vi "Turn (Gyro)(SubVI).vi"(7 "Ang S Up":dbl, 9 "AutoX":dbl, 10 "GyroRef":string="My Gyro RefNum", 11 "DriveMotorRefNum":string="RobotDrive") -> (3 "String":string)   [LabVIEW 2017]
uses:
  <vilib>/Rock Robotics/WPI/SafetyOutput/WPI_SafetyOutputConfigMenu.ctl
  <vilib>/Rock Robotics/WPI/Utilities/WPI_GetSetVariantRefNum.vi
  Robot Global Data.vi
  <vilib>/Rock Robotics/WPI/RobotDrive/WPI_RobotDriveArcadeDrive_Standard(NoSaturation).vi
  <vilib>/Rock Robotics/WPI/RobotDrive/WPI_RobotDriveSafetyCheck.vi
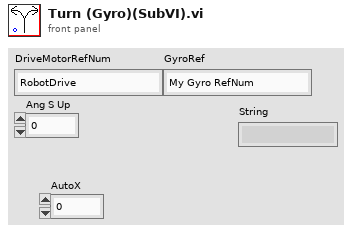
[diagram p1: front panel]
types:
  T1 = typedef "WPI_SafetyOutputConfigMenu.ctl" = enum16{"Enable", "Disable"}
  T2 = typedef "WPI_RobotDriveDevRef.ctl" = cluster{"DevStatus":errorcluster, "Motors[]":T3[], "Square Inputs":bool, "Max Output":dbl}
  T3 = typedef "WPI_MotorControlDeviceRef.ctl" = cluster{"DeviceStatus":errorcluster, "Type":T4, "PWM":cluster{"PWM Channel":T5, "DeadBand":T6}, "CAN":cluster{"Device Number":u8, "SetOutput VI Ref":variant, "GetOutput VI Ref":variant, "Enable VI Ref":variant, "Disable VI Ref":variant, "Data":variant}, "Invert":bool, "DIO PWM":cluster{"PWM \"Enable\" Channel":T5, "DIOChannel":T7, "PWM Rate":dbl}}
  T4 = typedef "WPI_MotorControlType.ctl" = enum16{"PWM", "CAN", "DIO PWM"}
  T5 = typedef "FPGA_DIOPWMChannel.ctl" = enum8{"PWM 0", "PWM 1", "PWM 2", "PWM 3", "PWM 4", "PWM 5", "PWM 6", "PWM 7", "PWM 8", "PWM 9", "PWM MXP 0", "PWM MXP 1", "PWM MXP 2", "PWM MXP 3", "PWM MXP 4", "PWM MXP 5", "PWM MXP 6", "PWM MXP 7", "PWM MXP 8", "PWM MXP 9", "Invalid"}
  T6 = typedef "WPI_PWMDeadband.ctl" = cluster{"Name":string, "maxPositivePwm":i32, "minPositivePwm":i32, "centerPwm":i32, "maxNegativePwm":i32, "minNegativePwm":i32, "angularRange":u16}
  T7 = typedef "FPGA_DIOChannel.ctl" = enum8{"DIO 0", "DIO 1", "DIO 2", "DIO 3", "DIO 4", "DIO 5", "DIO 6", "DIO 7", "DIO 8", "DIO 9", "DIO MXP 0", "DIO MXP 1", "DIO MXP 2", "DIO MXP 3", "DIO MXP 4", "DIO MXP 5", "DIO MXP 6", "DIO MXP 7", "DIO MXP 8", "DIO MXP 9", "DIO MXP 10", "DIO MXP 11", "DIO MXP 12", "DIO MXP 13", "DIO MXP 14", "DIO MXP 15", "SPI Port CS1", "SPI Port CS2", "SPI Port CS3", "SPI Port MISO", "SPI Port MOSI", "Invalid"}
  T8 = typedef "WPI_GyroDevRef.ctl" = cluster{"DevStatus":errorcluster, "Analog Channel":T9, "Gain (VoltsPerDegree/Second)":dbl, "Gyro Type":enum16{"Analog", "XRS450"}, "Handle":i32, "SPI Bus":T10, "Device Found":bool, "Sample Rate":dbl, "Calibrate On Open":bool, "Offset":dbl}
  T9 = typedef "FPGA_AIChannel.ctl" = enum8{"AI 0", "AI 1", "AI 2", "AI 3", "AI MXP 0", "AI MXP 1", "AI MXP 2", "AI MXP 3", "Invalid"}
  T10 = typedef "spi_bus.ctl" = enum16{"SPI On-Board, CS0", "SPI On-Board, CS1", "SPI On-Board, CS2", "SPI On-Board, CS3", "SPI MXP", "Invalid"}
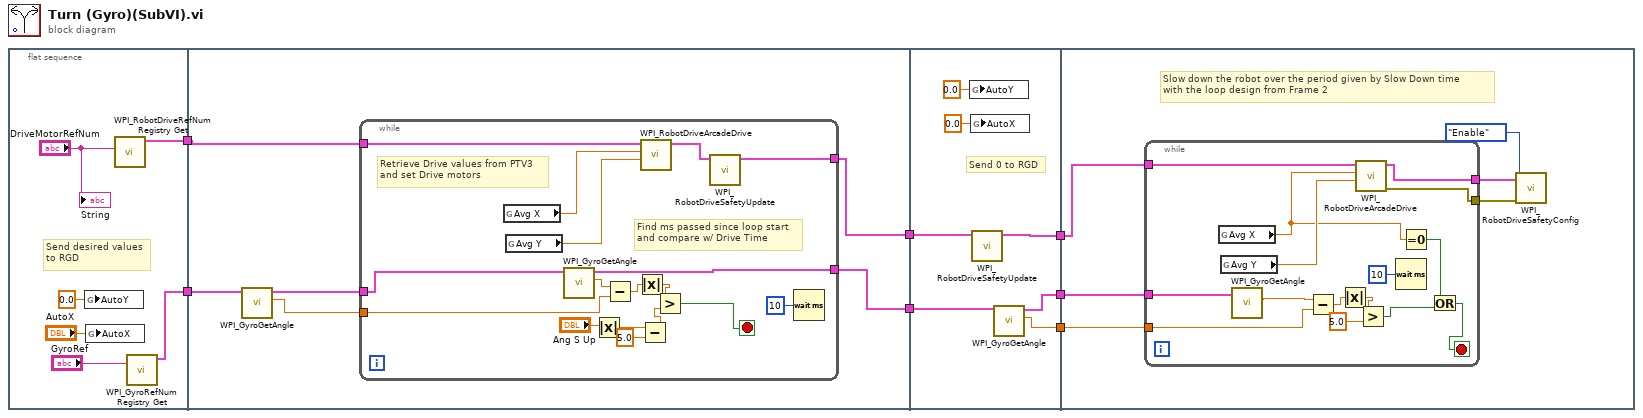
[diagram p0: block diagram]
diagram:
  n1 = flat-sequence {
    tunnel: [w13] -> w7
    tunnel: [w8] -> w4
    tunnel: w7 -> [w19]
    tunnel: [w18] -> w6
    tunnel: w4 -> [w17]
    tunnel: [w15] -> w3
    tunnel: [w42] -> w5
    tunnel: w6 -> [w43]
    tunnel: w3 -> [w39]
    tunnel: [w38] -> w2
    tunnel: [w37] -> w1
    tunnel: w5 -> [w49]
    tunnel: w2 -> [w45]
    tunnel: w1 -> [w44]
    frame #0 {
      # "Send desired values\nto RGD"
      n2 = global write "Robot Global Data.vi" "AutoY"(0.0 ("AutoY")) -> ()
      n3 = global write "Robot Global Data.vi" "AutoX"("AutoX") -> ()
      n4 = call <vilib>:"WPI_RobotDriveRefNum Registry Get.vi"("refnum name"="DriveMotorRefNum") -> ("RobotDriveDevRef"=w13:T2)  [unwired: 9 in, 1 out]
      n5 = call <vilib>:"WPI_GyroRefNum Registry Get.vi"("refnum name"="GyroRef") -> ("GyroDevRef"=w8:T8)  [unwired: 9 in, 1 out]
      "String" <- "DriveMotorRefNum"
    }
    frame #1 {
      n6 = call <vilib>:"WPI_GyroGetAngle.vi"("GyroDevRef"=w17) -> ("Angle"=w16:dbl, "GyroDevRef"=w14:T8)  [unwired: 7 in, 2 out]
      n7 = while {
        tunnel: w19 -> [w34]
        tunnel: [w31] -> w18
        tunnel: w14 -> [w30]
        tunnel: w16 -> [w28]
        tunnel: [w27] -> w15
        stop <- w33 stop-if-true
        # "Retrieve Drive values from PTV3\nand set Drive motors"
        # "Find ms passed since loop start\nand compare w/ Drive Time"
        n8 = global read "Robot Global Data.vi" "Avg X"() -> (w36:dbl)
        n9 = global read "Robot Global Data.vi" "Avg Y"() -> (w35:dbl)
        n10 = call <vilib>:"WPI_GyroGetAngle.vi"("GyroDevRef"=w30) -> ("Angle"=w29:dbl, "GyroDevRef"=w27:T8)  [unwired: 7 in, 2 out]
        n11 = Absolute Value(x="Ang S Up") -> (abs(x)=w22:dbl)
        n12 = Subtract(x=w29, y=w28) -> (x-y=w25:dbl)
        n13 = Absolute Value(x=w25) -> (abs(x)=w24:dbl)
        n14 = Subtract(x=w22, y=5.0) -> (x-y=w20:dbl)
        n15 = call-poly <vilib>:"WPI_RobotDriveArcadeDrive.vi"("Y axis value"=w35, "X axis value"=w36, "RobotDriveDevRef"=w34) -> ("RobotDriveDevRef"=w32:T2)  [unwired: 6 in, 2 out]
        n16 = Greater?(x=w24, y=w20) -> (0:w33:bool)
        n17 = call <vilib>:"WPI_RobotDriveSafetyUpdate.vi"("RobotDriveDevRef"=w32) -> ("RobotDriveDevRef"=w31:T2)  [unwired: 1 in, 9 out]
        n18 = Wait (ms)(milliseconds to wait=u32 10) -> ()  [unwired: 1 out]
      }
    }
    frame #2 {
      # "Send 0 to RGD"
      n19 = global write "Robot Global Data.vi" "AutoY"(0.0 ("AutoY")) -> ()
      n20 = global write "Robot Global Data.vi" "AutoX"(0.0 ("AutoX")) -> ()
      n21 = call <vilib>:"WPI_RobotDriveSafetyUpdate.vi"("RobotDriveDevRef"=w43) -> ("RobotDriveDevRef"=w42:T2)  [unwired: 1 in, 9 out]
      n22 = call <vilib>:"WPI_GyroGetAngle.vi"("GyroDevRef"=w39) -> ("Angle"=w38:dbl, "GyroDevRef"=w37:T8)  [unwired: 7 in, 2 out]
    }
    frame #3 {
      # "Slow down the robot over the period given by Slow Down time\nwith the loop design from Frame 2"
      n23 = while {
        tunnel: w49 -> [w63]
        tunnel: [w62] -> w48
        tunnel: [w61] -> w47
        tunnel: w45 -> [w56]
        tunnel: w44 -> [w55]
        stop <- w50 stop-if-true
        n24 = global read "Robot Global Data.vi" "Avg X"() -> (w53:dbl)
        n25 = global read "Robot Global Data.vi" "Avg Y"() -> (w64:dbl)
        n26 = call <vilib>:"WPI_GyroGetAngle.vi"("GyroDevRef"=w55) -> ("Angle"=w54:dbl)  [unwired: 7 in, 3 out]
        n27 = Subtract(x=w54, y=w56) -> (x-y=w59:dbl)
        n28 = Absolute Value(x=w59) -> (abs(x)=w60:dbl)
        n29 = call-poly <vilib>:"WPI_RobotDriveArcadeDrive.vi"("Y axis value"=w64, "X axis value"=w53, "RobotDriveDevRef"=w63) -> ("error out"=w61:errorcluster, "RobotDriveDevRef"=w62:T2)  [unwired: 6 in, 1 out]
        n30 = Greater?(x=w60, y=5.0) -> (0:w51:bool)
        n31 = Wait (ms)(milliseconds to wait=u32 10) -> ()  [unwired: 1 out]
        n32 = Equal To 0?(x=w53) -> (x = 0?=w52:bool)
        n33 = Or(x=w52, y=w51) -> (x .or. y?=w50:bool)
      }
      n34 = call <vilib>:"WPI_RobotDriveSafetyConfig.vi"("error in (no error)"=w47, "mode"=WPI_SafetyOutputConfigMenu."Enable", "RobotDriveDevRef"=w48) -> ()  [unwired: 7 in, 2 out]
    }
  }
